vi "Error Log.vi"(8 "error in (no error)":errorcluster) -> ()   [LabVIEW 2018]
doc: "This VI will log all errors to file with a description of the error\nthe level of the error\nthe time and date that the error occurred\nthe station step and time at which the error occurred.\n\nIf there is no error, this VI will do nothing"
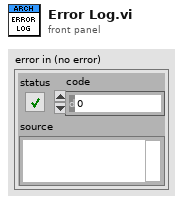
[diagram p1: front panel]
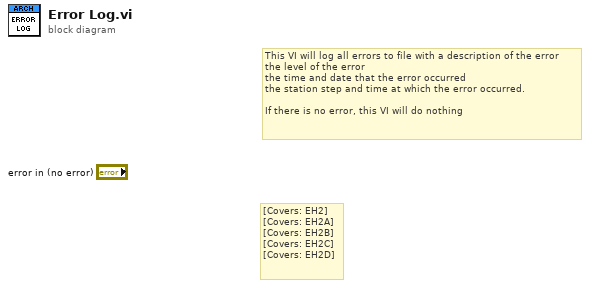
[diagram p0: block diagram]
diagram:
  # "[Covers: EH2]\n[Covers: EH2A]\n[Covers: EH2B]\n[Covers: EH2C]\n[Covers: EH2D]"
  # "This VI will log all errors to file with a description of the error\nthe level of the error\nthe time and date that the error occurred\nthe station step and time at which the error occurred.\n\nIf there is no error, this VI will do nothing"
